vi "TWM Calculate.vi"(7 "session info path":path=path "D:/martin/WAC/WACsw - github/control_software/Filter function meter/Template/Example of FF meter template_data/FF_calibration_template_line_0010/session.info", 8 "error in (no error)":errorcluster, 11 "Common properties":T1={"Measurement status ref"=refnum, "TWM Status ref"=refnum, "Abort ref"=refnum, "Skip waiting ref"=refnum, "GNU Octave path"=path "C:/Program Files/GNU Octave/Octave-6.2.0/mingw64/bin", "TWM+QWTB path"=path "C:/Users/labina/Desktop/TWM-1.8.7.0-full/octprog", "lvlib path"=path "D:/martin/WAC/WACsw - github/control_software/Filter function meter/external libraries/GOLPI 0.7.3.1 source distribution LV 20.0 32 bit/lv_proc.dll", "TWM pipe"="\\\\.\\pipe\\TWM:server", "PJVS status ref"=refnum, "WAC path"=path ""}) -> (0 "error out":errorcluster)   [LabVIEW 2020]
doc: "Starts and waits for QWTB calculation."
uses:
  Type definitions/Common properties.ctl
  Globals for GOLPI.vi
  external libraries/GOLPI 0.7.3.1 source distribution LV 20.0 32 bit/GOLPI library.lvlib
panel:
  out "command\n(for debug)":string="addpath('info'); addpath('qwtb'); qwtb_exec_algorithm('%s', 0, 1); disp('FINISHEDCR')"
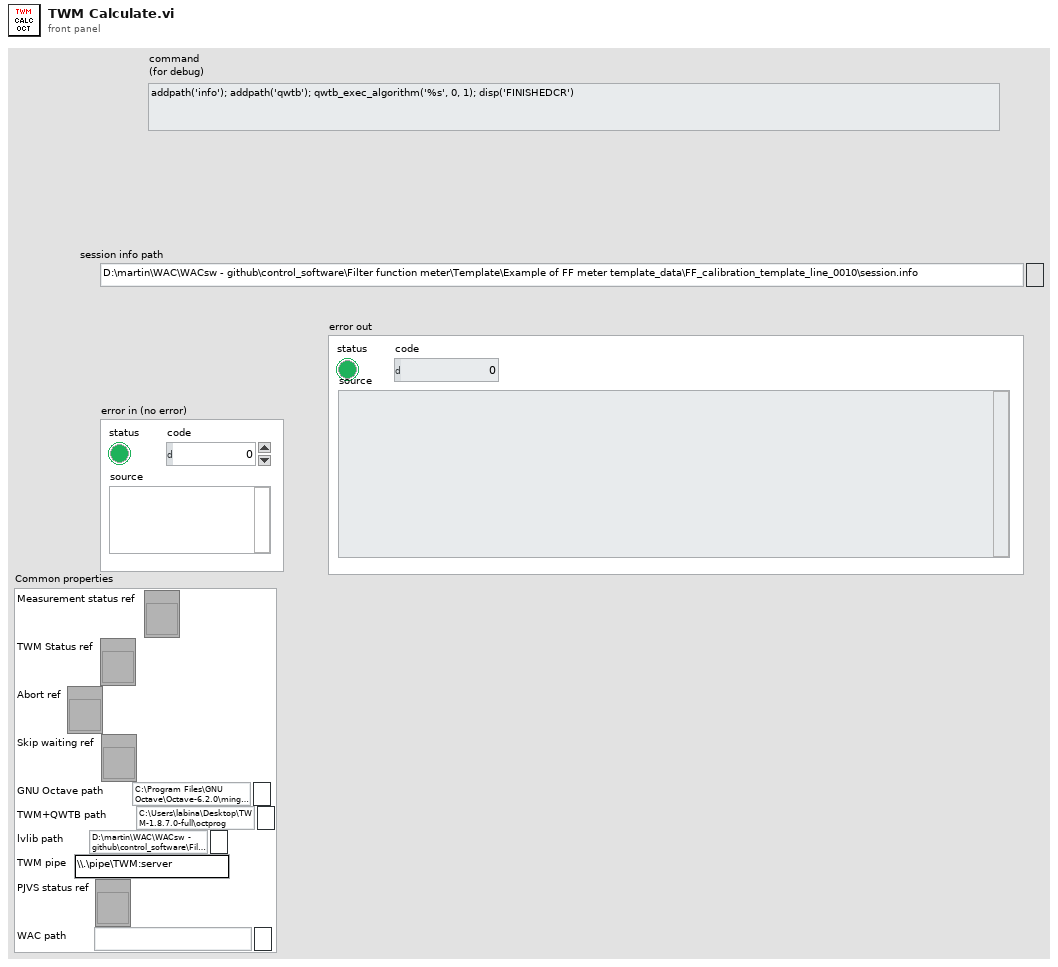
[diagram p1: front panel]
types:
  T1 = typedef "Common properties.ctl" = cluster{"Measurement status ref":refnum<vi>, "TWM Status ref":refnum<vi>, "Abort ref":refnum<vi>, "Skip waiting ref":refnum<vi>, "GNU Octave path":path, "TWM+QWTB path":path, "lvlib path":path, "TWM pipe":string, "PJVS status ref":refnum<vi>, "WAC path":path}
  T2 = typedef "GOLPI library.lvlib/GOLPI reference Type Def.ctl" = cluster{"pipe handle":T3, "fast read timeout [ms]":u32, "fast read settle time [ms]":u32, "fast read to multiple [ms]":u32, "max elements per input line":u32, "slow read timeout [ms]":u32, "stdin double format specifier":string, "max elements per stdout output column":u32, "console mode bitstream":bool, "bitstream first read timeout [ms]":u32, "bitstream read timeout [ms]":u32, "struct transfer possible":bool, "matlab mode":bool}
  T3 = typedef "LV Process library.lvlib/Pipe Handle.ctl" = cluster{"lv_proc.dll file path":path, "process instance handle":u32[], "debug mode":bool, "debug data":cluster{"time":timestamp, "stdin":bool, "data":string}[]}
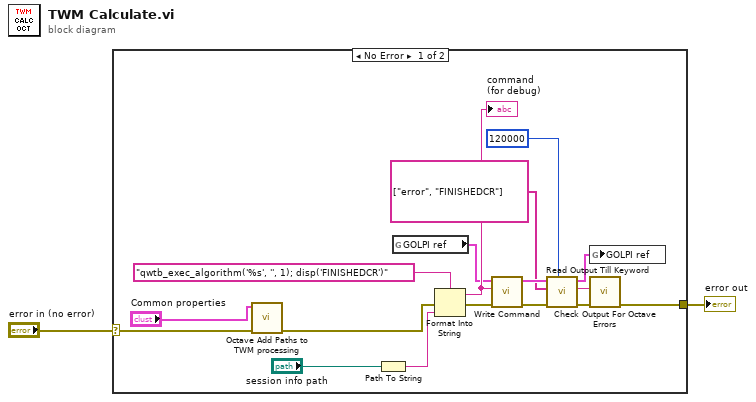
[diagram p0: block diagram]
diagram:
  n1 = case shown="No Error" "error in (no error)" {
    selector: "error in (no error)" -> [w4 w20]
    tunnel: [w6 w20] -> w2
    frame No Error {
      n2 = call "Octave Add Paths to TWM processing.vi"("error in (no error)"=w4, "Common properties"="Common properties") -> ("error out"=w3:errorcluster)  [unwired: 9 in]
      n3 = Path To String(path="session info path") -> (string=w17:string)
      n4 = global read "Globals for GOLPI.vi" "GOLPI ref"() -> (w10:T2)
      n5 = Format Into String(format string="qwtb_exec_algorithm('%s', '', 1); disp('FINISHEDCR')", error in=w3, w17) -> (resulting string=w11:string, error out=w16:errorcluster)  [unwired: 1 in]
      "command\n(for debug)" <- w11
      n6 = call "Write Command.vi"("error in"=w16, "command"=w11, "GOLPI ref. in"=w10) -> ("error out"=w15:errorcluster, "GOLPI ref. out"=w14:T2)  [unwired: 7 in]
      n7 = call "Read Output Till Keyword.vi"("timeout [ms]"=u32 120000, "error in"=w15, "keywords"=string[] ["error", "FINISHEDCR"], "GOLPI ref. in"=w14) -> ("error out"=w8:errorcluster, "read buffer"=w7:string, "GOLPI ref. out"=w9:T2)  [unwired: 4 in, 1 out]
      n8 = global write "Globals for GOLPI.vi" "GOLPI ref"(w9) -> ()
      n9 = call "Check Output For Octave Errors.vi"("error in"=w8, "read buffer"=w7) -> ("error out"=w6:errorcluster)  [unwired: 9 in]
    }
    frame Error {
    }
  }
  "error out" <- w2
